vi "Variables Automo Global.vi"() -> ()   [LabVIEW 2015]
panel:
  in  "Feeder":bool
  in  "Disparar":bool
  in  "Auto-Aim":bool
  in  "Giro":dbl
  in  "Adelante/Atras":dbl
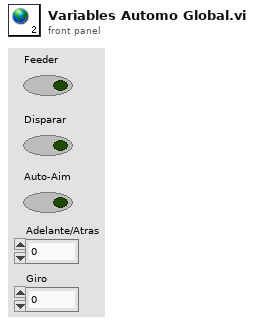
[diagram p1: front panel]
diagram:
